vi "BRig_RT__Case_Exp__UploadClosedLoop.vi"() -> ()   [LabVIEW 2014]
panel:
  out "size":i64
  out "path out":path
  out "error out":errorcluster
  out "output_val":u16
  out "output_idx":i32
  out "output_dataType":u8
  out "output_haveCmd":bool
  out "received":bool
  out "text":string
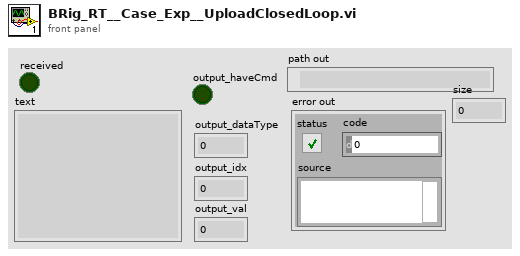
[diagram p1: front panel]
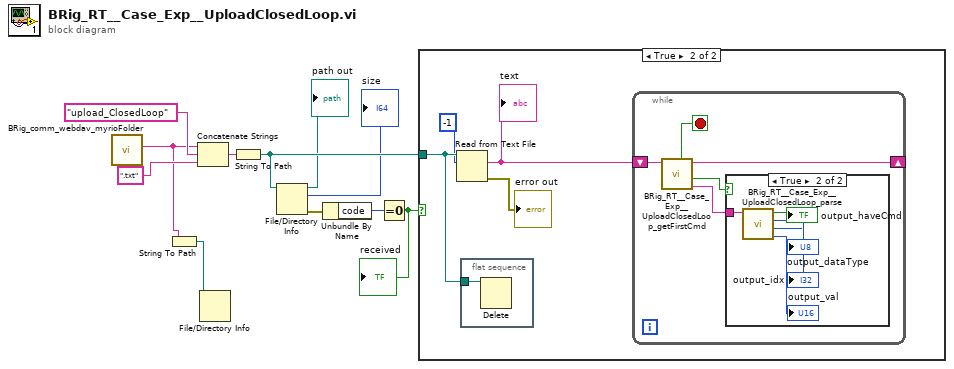
[diagram p0: block diagram]
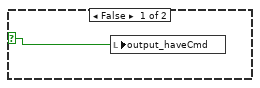
[diagram p2: hidden frame]
diagram:
  n1 = call "BRig_comm_webdav_myrioFolder.vi"() -> ("output_myrioFolder"=w4:string)  [unwired: 11 in]
  n2 = String To Path(string=w4) -> (path=w3:path)
  n3 = Concatenate Strings(w4, "upload_ClosedLoop" ("string"), ".txt" ("string")) -> (w11:string)
  n4 = File/Directory Info(path=w3) -> ()  [unwired: 1 in, 7 out]
  n5 = String To Path(string=w11) -> (path=w5:path)
  n6 = File/Directory Info(path=w5) -> (path out=→"path out":path, size=→"size":i64, error out=w8:errorcluster)  [unwired: 1 in, 4 out]
  n7 = Unbundle By Name(w8) -> ("code"=w7:i32)
  n8 = Equal To 0?(x=w7) -> (x = 0?=w6:bool)
  "received" <- w6
  n9 = case shown="True" w6 {
    selector: w6 -> [w12 _]
    tunnel: w5 -> [_ w16]
    frame False {
      n10 = local write "output_haveCmd"(w12) -> ()
    }
    frame True {
      n11 = Read from Text File(file (use dialog)=w16, count=-1) -> (text=w15:string, error out=→"error out":errorcluster)  [unwired: 2 in, 2 out]
      "text" <- w15
      n12 = flat-sequence {
        tunnel: w16 -> [w27]
        frame #0 {
          n13 = Delete(path (use dialog)=w27) -> ()  [unwired: 4 in, 3 out]
        }
      }
      n14 = while {
        shift-right: [w19] -> _
        shift-left: w15 -> [w21]
        stop <- w20 stop-if-true
        n15 = call "BRig_RT__Case_Exp__UploadClosedLoop_getFirstCmd.vi"("input_str"=w21) -> (0:"output_cmd"=w17:string, 1:"output_cmd"=w18:bool, "output_str"=w19:string, "output_abort"=w20:bool)  [unwired: 7 in]
        n16 = case shown="True" w18 {
          tunnel: w17 -> [_ w26]
          frame False {
          }
          frame True {
            n17 = call "BRig_RT__Case_Exp__UploadClosedLoop_parse.vi"("input_strCmd"=w26) -> ("output_val"=→"output_val":u16, "output_idx"=→"output_idx":i32, "output_dataType"=→"output_dataType":u8, "output_haveCmd"=→"output_haveCmd":bool)  [unwired: 7 in]
          }
        }
      }
    }
  }
